vi "Read SA Pin.vi"(8 "error in (no error)":errorcluster, 11 "LTE_SEM in":refnum<class "NR_SEM.lvclass">) -> (0 "error out":errorcluster, 2 "SA Pin":string, 3 "LTE_SEM out":refnum<class "NR_SEM.lvclass">)   [LabVIEW 2018, in "SeqAuto Evaluations.lvlib" / "NR_SEM.lvclass"]
uses:
  NR_SEM.lvclass
  NR_SEM.lvclass/NR_SEM.ctl
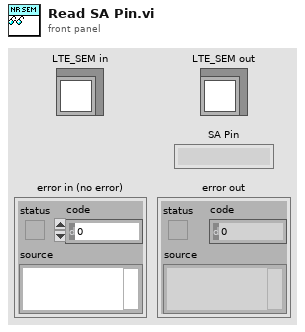
[diagram p1: front panel]
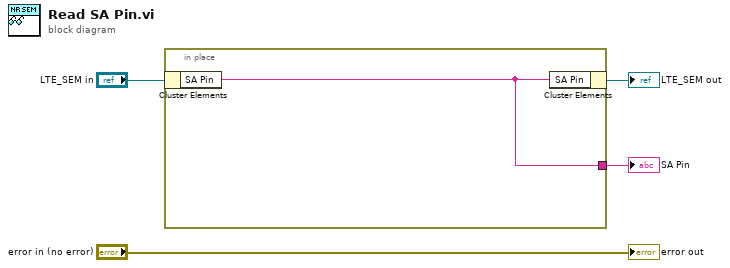
[diagram p0: block diagram]
diagram:
  n1 = in-place {
    in-place-border: [w5] -> w1
    n2 = in-place-cluster #1("LTE_SEM in") -> ("SA Pin"=w5:string)
    n3 = in-place-cluster #1("SA Pin"=w5) -> (→"LTE_SEM out":refnum<class "NR_SEM.lvclass">)
  }
  "SA Pin" <- w1
  "error out" <- "error in (no error)"
